vi "Create Lookup Table.vi"(8 "error in (no error)":errorcluster) -> (0 "error out":errorcluster, 3 "LookupTable Reference":refnum<data-value>)   [LabVIEW 2020, in "LookupTable.lvlib" / "LookupTable.lvclass"]
uses:
  <vilib>/gpm_packages/@cs/lookup-table/Source/LookupTable/LookupTable.lvclass
  <vilib>/gpm_packages/@cs/lookup-table/Source/LookupTable/LookupTable.lvclass/LookupTable.ctl
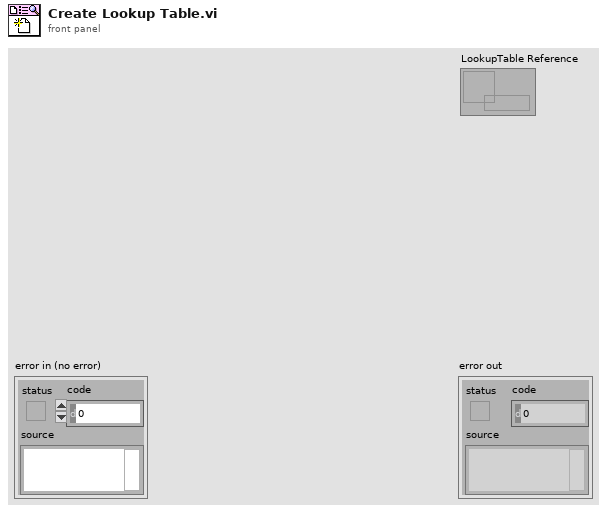
[diagram p1: front panel]
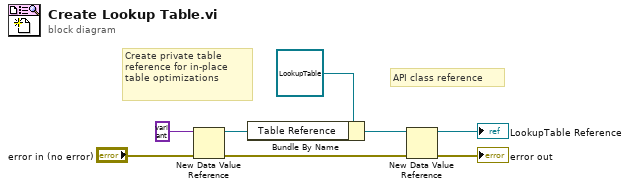
[diagram p0: block diagram]
diagram:
  # "API class reference"
  # "Create private table\nreference for in-place\ntable optimizations"
  n1 = New Data Value Reference(data value=variant, error in="error in (no error)") -> (data value reference=w3:refnum<data-value>, error out=w1:errorcluster)
  n2 = Bundle By Name(cluster=refnum<class "LookupTable.lvclass"> refnum, "Table Reference"=w3) -> (w4:refnum<class "LookupTable.lvclass">)
  n3 = New Data Value Reference(data value=w4, error in=w1) -> (data value reference=→"LookupTable Reference":refnum<data-value>, error out=→"error out":errorcluster)
